vi "AgNA_Wait For Sweep Complete.vi"(8 "error in (no error)":errorcluster {"code" format="%.0x"}, 9 "MaxTimeMilliseconds":i32 format="%.0g", 10 "Channel":string, 11 "instrument handle":refnum<k15>) -> (0 "error out":errorcluster {"code" format="%.0x"}, 3 "instrument handle out":refnum<k15>)   [LabVIEW 2015]
uses:
  <instrlib>/Agilent NA/Agilent NA.lvlib
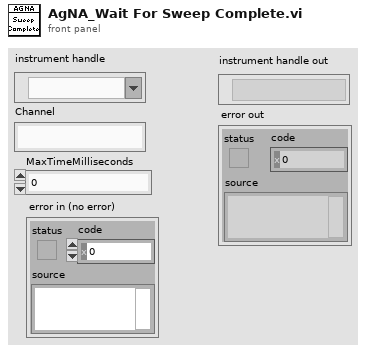
[diagram p1: front panel]
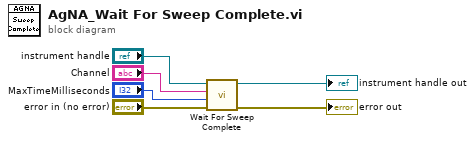
[diagram p0: block diagram]
diagram:
  n1 = call <instrlib>:"Wait For Sweep Complete.vi"("error in (no error)"="error in (no error)", "MaxTimeMilliseconds"="MaxTimeMilliseconds", "Channel"="Channel", "instrument handle"="instrument handle") -> ("error out"=→"error out":errorcluster, "instrument handle out"=→"instrument handle out":refnum<k15>)  [unwired: 6 in]
